vi "Init.vi"(8 "error in (no error)":errorcluster, 10 "Test Group Data":T1) -> (0 "error out":errorcluster, 3 "data value reference":refnum<data-value>)   [LabVIEW 2016, in "Test Group Manager.lvlib" / "Test Group.lvclass"]
uses:
  Test Group.lvclass
  Test Group.lvclass/Test Group.ctl
  Write Test Group Data.vi
  Write DPD Initialized.vi
  Write Input Power Initialized.vi
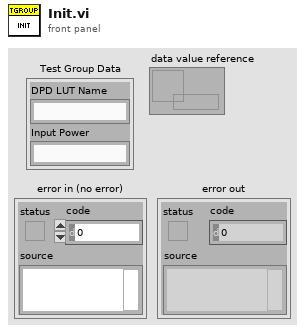
[diagram p1: front panel]
types:
  T1 = cluster{"DPD LUT Name":string, "Input Power":string}
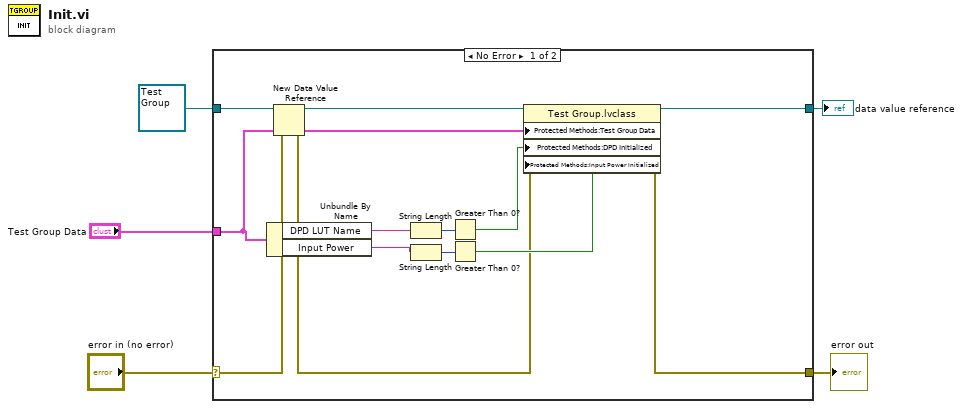
[diagram p0: block diagram]
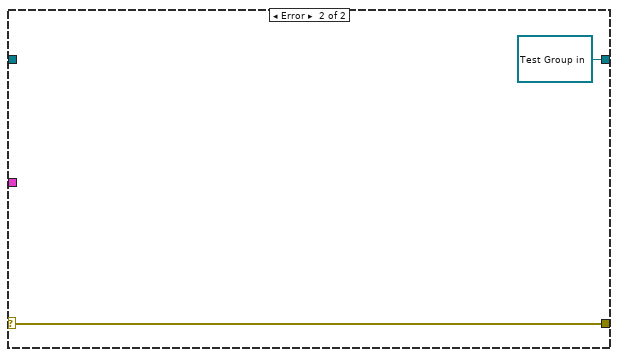
[diagram p2: hidden frame]
diagram:
  n1 = case shown="No Error" "error in (no error)" {
    selector: "error in (no error)" -> [w18 w20]
    tunnel: [w17 w20] -> w4
    tunnel: [w16 refnum<data-value> refnum ("data value reference")] -> w1
    tunnel: refnum<class "Test Group.lvclass"> refnum ("Test Group in") -> [w7 _]
    tunnel: "Test Group Data" -> [w15 _]
    frame No Error {
      n2 = Unbundle By Name(w15) -> ("DPD LUT Name"=w14:string, "Input Power"=w11:string)
      n3 = New Data Value Reference(data value=w7, error in=w18) -> (data value reference=w6:refnum<data-value>, error out=w8:errorcluster)
      n4 = String Length(string=w14) -> (length=w13:i32)
      n5 = String Length(string=w11) -> (length=w12:i32)
      n6 = Greater Than 0?(x=w13) -> (x > 0?=w10:bool)
      n7 = Greater Than 0?(x=w12) -> (x > 0?=w9:bool)
      n8 = property class="Test Group.lvclass"(reference=w6, error in=w8, "Protected Methods:Test Group Data"=w15, "Protected Methods:DPD Initialized"=w10, "Protected Methods:Input Power Initialized"=w9) -> (reference out=w16:refnum<data-value>, error out=w17:errorcluster)
    }
    frame Error {
    }
  }
  "error out" <- w4
  "data value reference" <- w1
